vi "LiftArm Calibration.vi"(11 "NXT/EV3":T1) -> (3 "NXT/EV3 2":T1)   [LabVIEW 2016]
uses:
  <vilib>/NXT/Subs/LVHSConnector.ctl
  <vilib>/NXT/LegoClasses/BrickReference/BrickReference.lvclass
  <vilib>/NXT/Block Support/NXT_OutputPort.ctl
  <vilib>/NXT/NXTIO Xnodes/NXTIONodeSubVIs/NXTMotorRunDistance.vi
  <vilib>/NXT/NXTIO Xnodes/AddressXNode/NXTIOAddress.xnode
  <vilib>/NXT/NXTIO Xnodes/NXTIOXNode/NXTIO.xnode
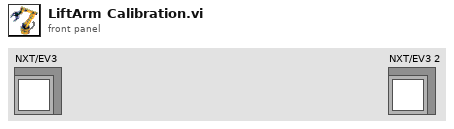
[diagram p1: front panel]
types:
  T1 = typedef "LVHSConnector.ctl" = refnum<class "BrickReference.lvclass">
  T2 = typedef "NXT_OutputPort.ctl" = u8
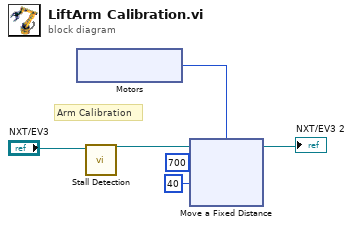
[diagram p0: block diagram]
diagram:
  # "Arm Calibration"
  n1 = xnode "Motors"() -> ("Motor"=w3:T2)
  n2 = call "Stall Detection.vi"("NXT/EV3"="NXT/EV3") -> ("NXT/EV3"=w4:T1)  [unwired: 10 in]
  n3 = xnode "Move a Fixed Distance"("Speed 1"=i8 40, "Distance 1"=700, "Motors"=w3, "NXT/EV3"=w4) -> ("NXT/EV3"=→"NXT/EV3 2":T1)
